vi "Login.vi"(8 "error in (no error)":errorcluster, 11 "Login Input":T2) -> (0 "error out":errorcluster, 3 "Login Output":T1)   [LabVIEW 2023]
doc: "This program is used for LogIn/LogOut functions. this is selected by setting mode 1/2 and by entering all other fields (Equipment number = Sttaion number, and MES user)\nPossible errors :\nE020 SAP user data not found for logged in user [{0}]. -> There is no SAP user associated with the login user. \nE021 User data not found for logged in user [{0}]. -> The logged-in user is not registered in MES.\nE022 Equipment [{0}] is in running. -> User is already logged in\nE023 Equipment [{0}] is in stop. -> User is already Logged off \nE024 Undefined mode [{0}] has been set. -> currently only possible modes are 1 for Log In and 2 for Log out"
uses:
  <userlib>/WebService/_CheckUserAndEquipmentStatusService/CheckUserAndEquipmentStatusService.lvlib
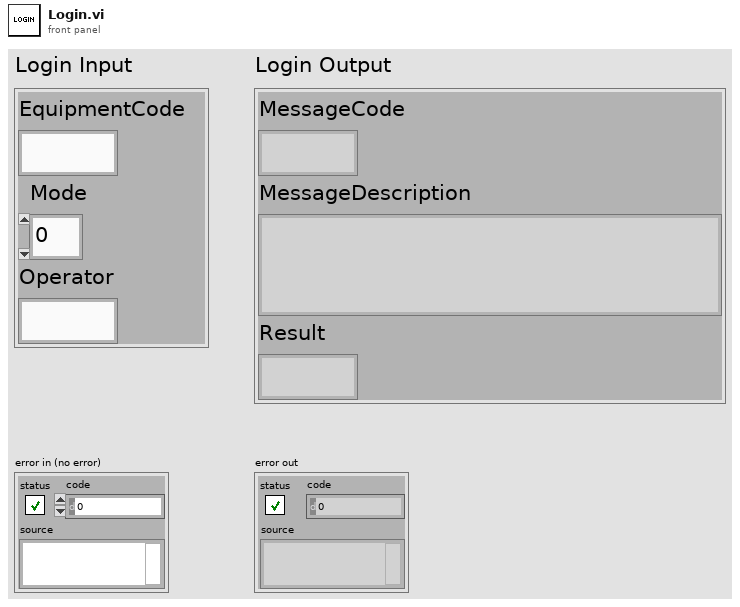
[diagram p1: front panel]
types:
  T1 = cluster{"MessageCode":string, "MessageDescription":string, "Result":string}
  T2 = cluster{"EquipmentCode":string, "Mode":i32, "Operator":string}
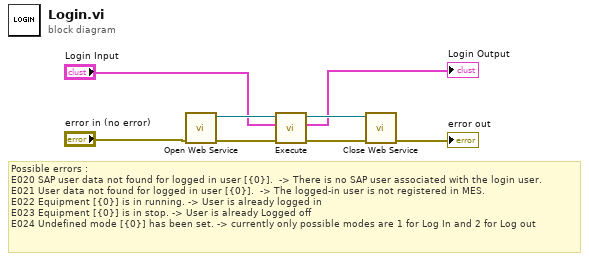
[diagram p0: block diagram]
diagram:
  # "Possible errors :\nE020 SAP user data not found for logged in user [{0}].  -> There is no SAP user associated with the login user. \nE021 User data not found for logged in user [{0}].  -> The logged-in user is not registered in MES.\nE022 Equipment [{0}] is in running. -> User is already logged in\nE023 Equipment [{0}] is in stop. -> User is already Logged off \nE024 Undefined mode [{0}] has been set. -> currently only possible modes are 1 for Log In and 2 for Log out"
  n1 = call <userlib>:"Open Web Service.vi"("error in (no error)"="error in (no error)") -> ("error out"=w6:errorcluster, "CheckUserAndEquipmentStatusService refnum"=w7:refnum<k24>)  [unwired: 9 in]
  n2 = call <userlib>:"Execute.vi"("error in (no error)"=w6, ".NET:CheckUserAndEquipmentStatusService.UserAndEquipmentStatusRequest"="Login Input", "CheckUserAndEquipmentStatusService refnum"=w7) -> ("error out"=w3:errorcluster, ".NET:CheckUserAndEquipmentStatusService.CommonResponse"=→"Login Output":T1, "CheckUserAndEquipmentStatusService refnum out"=w4:refnum<k24>)  [unwired: 6 in]
  n3 = call <userlib>:"Close Web Service.vi"("error in (no error)"=w3, "CheckUserAndEquipmentStatusService refnum"=w4) -> ("error out"=→"error out":errorcluster)  [unwired: 9 in]
